vi "Write Name Dependecy.vi"(8 "error in (no error)":errorcluster, 10 "Name Dependecy":i32, 11 "Listbox TBDT in":refnum<class "Listbox TBDT.lvclass">) -> (0 "error out":errorcluster, 3 "Listbox TBDT out":refnum<class "Listbox TBDT.lvclass">)   [LabVIEW 2013, in "Table Manager.lvlib" / "Listbox TBDT.lvclass"]
uses:
  Listbox TBDT.lvclass
  Listbox TBDT.lvclass/Listbox TBDT.ctl
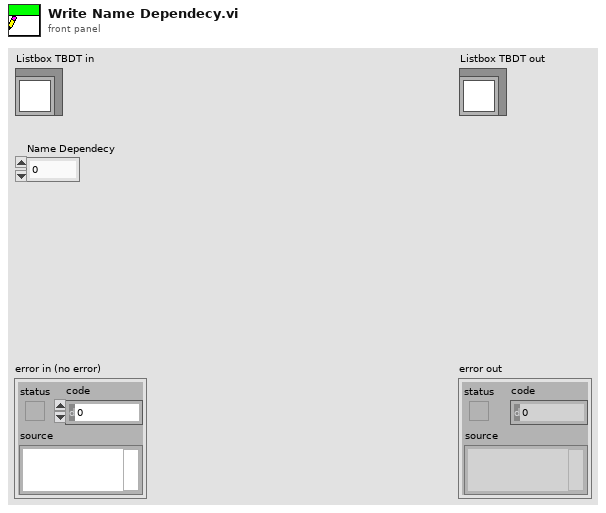
[diagram p1: front panel]
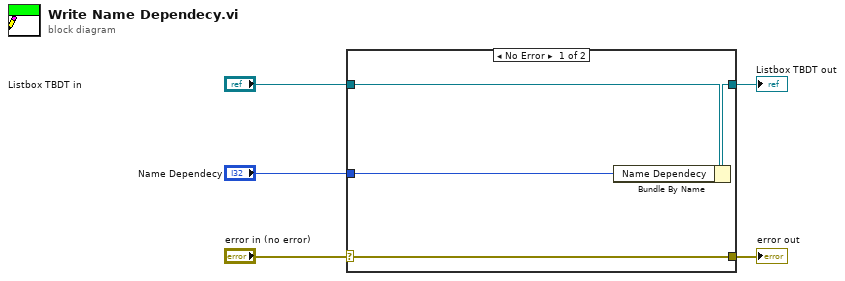
[diagram p0: block diagram]
diagram:
  n1 = case shown="No Error" "error in (no error)" {
    selector: "error in (no error)" -> [w9 w10]
    tunnel: [w9 w10] -> w4
    tunnel: [w7 w11] -> w2
    tunnel: "Listbox TBDT in" -> [w8 w11]
    tunnel: "Name Dependecy" -> [w6 _]
    frame No Error {
      n2 = Bundle By Name(cluster=w8, "Name Dependecy"=w6) -> (w7:refnum<class "Listbox TBDT.lvclass">)
    }
    frame Error {
    }
  }
  "error out" <- w4
  "Listbox TBDT out" <- w2
